vi "decode-sub33.vi"() -> ()   [LabVIEW 2010]
panel:
  out "x-y":u32
  in  "input string":string="B455"
  out "output data":i32
  out "数字 3":u32
  out "数字 2":u32
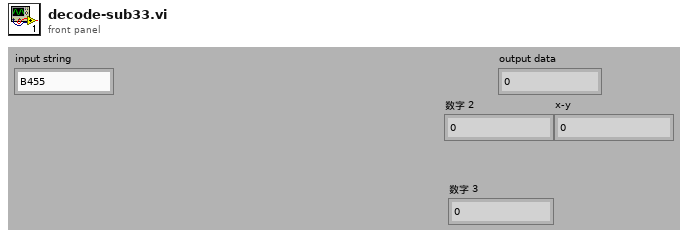
[diagram p1: front panel]
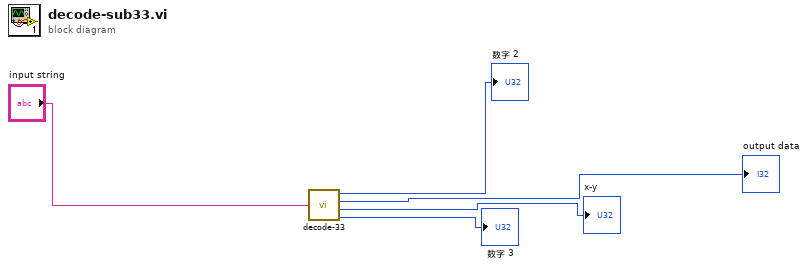
[diagram p0: block diagram]
diagram:
  n1 = call "decode-33.vi"("input string"="input string") -> ("数字 3"=→"数字 3":u32, "x-y"=→"x-y":u32, "output data"=→"output data":i32, "数字 2"=→"数字 2":u32)
